vi "Firmware.vi"() -> ()   [LabVIEW 2017]
uses:
  <vilib>/Platform/TimedLoop/XDataNode/timing_clust.ctl
  <vilib>/Platform/TimedLoop/XDataNode/nitl_modes.ctl
  <vilib>/Platform/TimedLoop/XDataNode/wakeup.ctl
  <instrlib>/_niInstr/FIFO Register Bus/v1/FPGA/niInstr FIFO Register Bus v1 FPGA.lvclass
  C:/Program Files (x86)/National Instruments/LabVIEW 2017/instr.lib/_niInstr/Instruction Framework/v1/FPGA/Interfaces/Instruction Producer/Instruction Producer.lvclass
  <instrlib>/_niInstr/Instruction Framework/v1/FPGA/Helper Classes/Single Address Space Collection/Single Address Space Collection.lvclass
  C:/Program Files (x86)/National Instruments/LabVIEW 2017/instr.lib/_niInstr/Instruction Framework/v1/FPGA/Interfaces/Address Space Collection/Address Space Collection.lvclass
  <vilib>/rvi/Emulation/niFpgaGetClockAttributes.vi
  <vilib>/rvi/Emulation/niFpgaSctlEmulationGetInTimedLoop.vi
  <vilib>/rvi/Emulation/niFpgaEmulationReportErrorSimple.vi
  <userlib>/_NI FLP Library/FPGA/outsideSCTL/FlpLib Multiply Shared Instance 2.vi
  <userlib>/_NI FLP Library/FPGA/outsideSCTL/FlpLib Add Shared Instance 2.vi
  <userlib>/_NI FLP Library/FPGA/outsideSCTL/FlpLib Subtract Shared Instance 2.vi
  <userlib>/_NI FLP Library/FPGA/outsideSCTL/FlpLib Greater Than Shared Instance 2.vi
  <vilib>/rvi/Emulation/niFpgaProcessEmulError.vi
  <userlib>/_NI FLP Library/FPGA/outsideSCTL/FlpLib Cosine Shared Instance 2.vi
  <vilib>/rvi/Emulation/niFpgaCriticalErrorInLSC.vi
  <userlib>/_NI FLP Library/addons/PowerElectronics/ABCtoAlphaBeta_3PhaseUnitaryMagnitude/FlpLib ABCtoAlphaBeta_3PhaseUnitaryMagnitude 0.vi
  <userlib>/_NI FLP Library/FPGA/outsideSCTL/FlpLib Sine & Cosine Shared Instance 0.vi
  <userlib>/_NI FLP Library/addons/PowerElectronics/AlphaBetaToDQ_noSine/FlpLib AlphaBetaToDQ_noSine 0.vi
  <vilib>/platform/TimedLoop/XDataNode/XDataNode.xnode
  <vilib>/NI/PowerElectronicsControl/ThreePhasePLL/FPGA/ThreePhasePLL.lvlib
  <instrlib>/_niInstr/Instruction Framework/v1/FPGA/Top Level Bus/Register Configuration/Register Configuration.lvclass
  <vilib>/Platform/TimedLoop/XDataNode/XDNodeRunTimeDep.lvlib
  <vilib>/NI/PowerElectronicsControl/ThreePhasePLL/FPGA/AddressSpace.lvclass
panel:
  in  "fifo reg bus ctrl 0":u32
  out "fifo reg bus status 0":u32
  out "fifo reg bus data 0":u64
  in  "PLL_Timing":u32=400
  out "PLLTimingActual":u32
  out "gridFrequency":sgl
  out "freq error":sgl
  out "theta error":sgl
  in  "ThreePhaseGenTiming":u32=400
  out "ThreePhaseGenActual":u32
  in  "dTGen":sgl=1e-05 format="%#_13g"
  in  "GenFreqRadPerSec":sgl=376.991 format="%#_13g"
  out "gridTheta":sgl
  out "A":sgl
  out "B":sgl
  out "C":sgl
  in  "gain":sgl=100.0
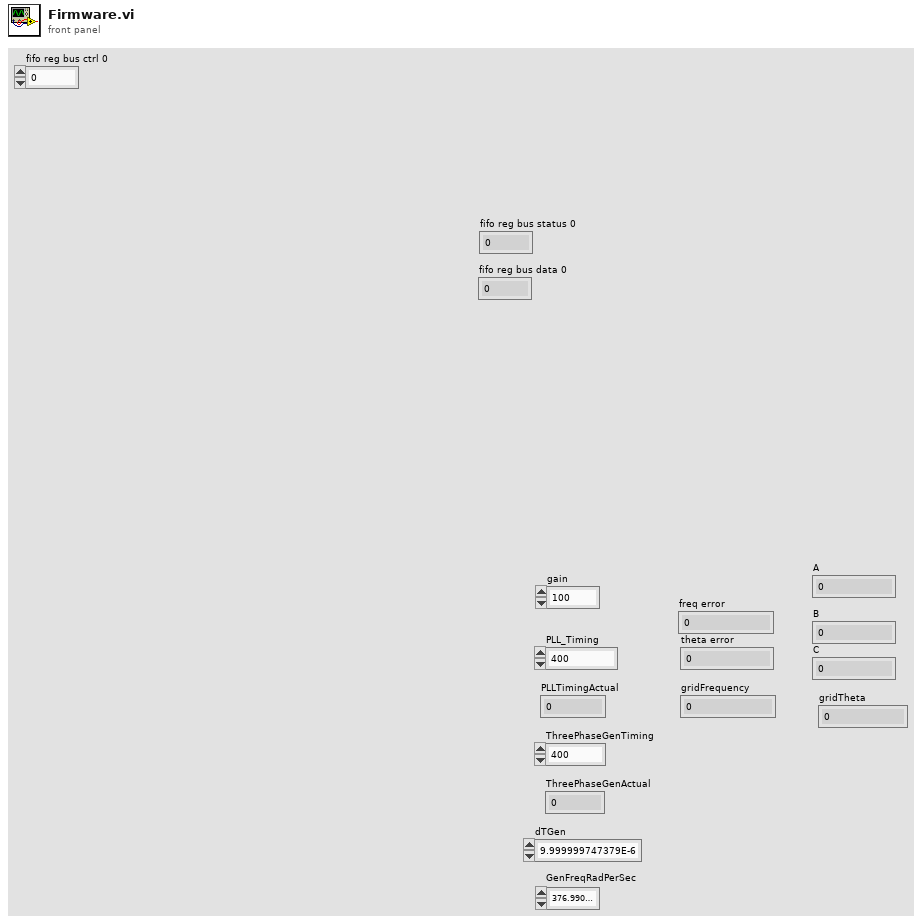
[diagram p1: front panel]
types:
  T1 = typedef "ThreePhasePLL.lvlib/registers.ctl" = cluster{"PLLGains":refnum<k21>, "PLLRange":refnum<k21>, "PLL_reset":refnum<k21>, "PLL_locked":refnum<k21>, "freqBoundaries":refnum<k21>, "expectedFreq":refnum<k21>, "lockDuration":refnum<k21>, "dT":refnum<k21>, "detectedFreq":refnum<k21>, "adjustTheta":refnum<k21>}
  T2 = typedef "XDNodeRunTimeDep.lvlib/timing_clust.ctl" = cluster{"Expected End [f-1]":u64, "Actual End [f-1]":u64, "Finished Late? [f-1]":bool, "Expected End [i-1]":u64, "Actual End [i-1]":u64, "Finished Late? [i-1]":bool, "Expected Start [i]":u64, "Actual Start [i]":u64, "Expected Start [f]":u64, "Actual Start [f]":u64, "Source Name":string, "Structure Name":string, "Period":i64, "Deadline":i64, "Offset":i64, "Start":i64, "Priority":i32, "Timeout":i32, "Mode":T3, "Wakeup Reason":T4, "Error":errorcluster, "Source Type":string, "Secondary Source Type":string, "Global End Time":u64, "Global Start Time":u64, "Frame Duration":u64, "Iteration Duration":u64, "Assigned CPU":i32, "I/O Scan Engine Mode":u32}
  T3 = typedef "XDNodeRunTimeDep.lvlib/nitl_modes.ctl" = enum32{"No Change", "Process missed periods, maintain original phase", "Discard missed periods, maintain original phase", "Process missed periods, ignore original phase", "Discard missed periods, ignore original phase"}
  T4 = typedef "XDNodeRunTimeDep.lvlib/wakeup.ctl" = enum32{"Normal", "Aborted", "Asynchronous wakeup", "Timing source error", "Timed loop error", "Timeout"}
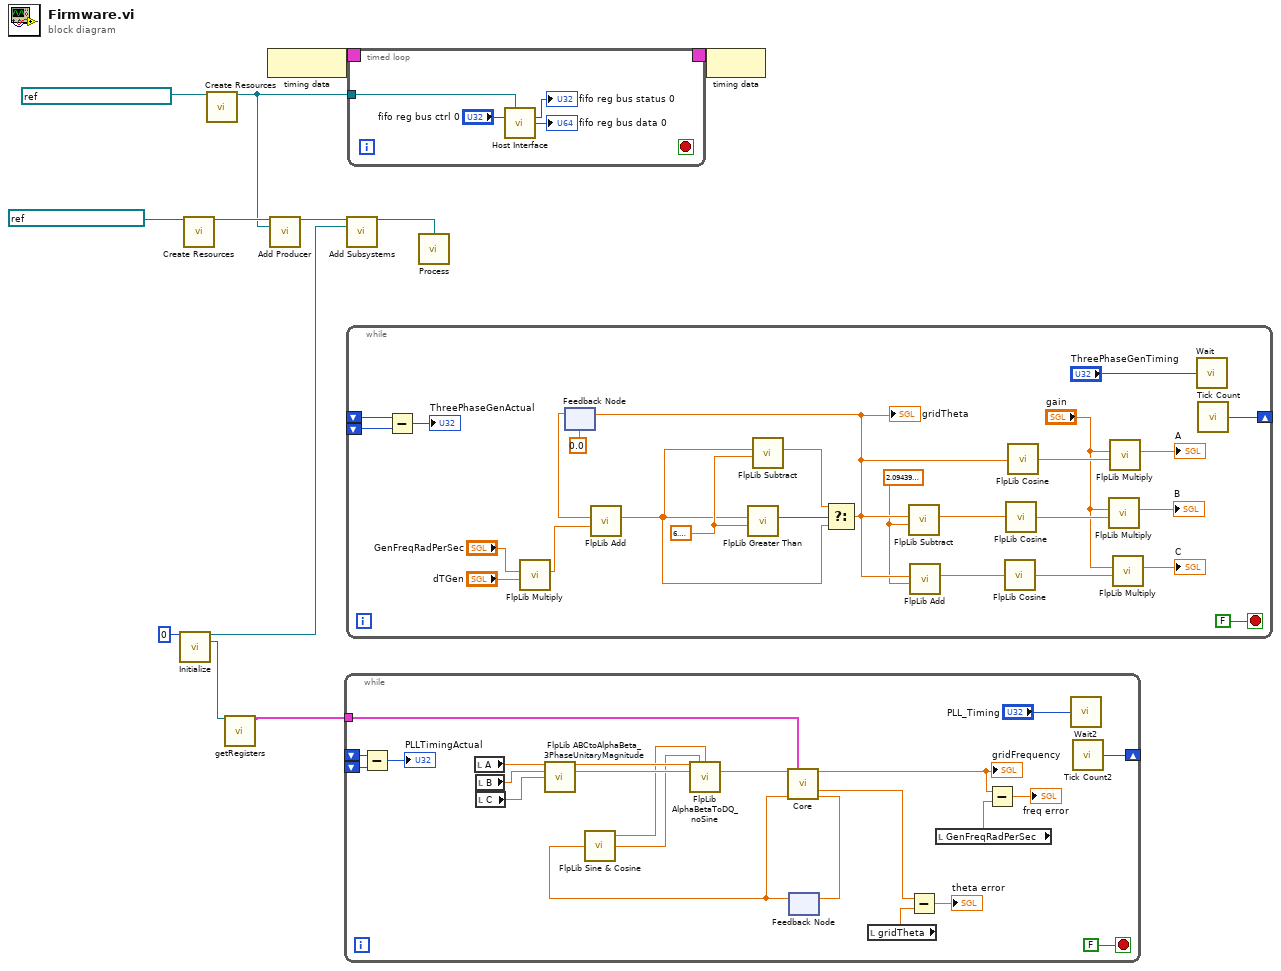
[diagram p0: block diagram]
diagram:
  n1 = call <vilib>:"Initialize.vi"("instance"=u8 0) -> ("subsysytem"=w2:refnum<class "Single Address Space Collection.lvclass">, "AddressSpace"=w4:refnum<class "AddressSpace.lvclass">)  [unwired: 13 in]
  n2 = call <instrlib>:"Create Resources.vi"("register clock"=refnum<k21> "40 MHz Onboard Clock") -> ("register configuration"=w8:refnum<class "Register Configuration.lvclass">)  [unwired: 14 in]
  n3 = call <instrlib>:"Create Resources.vi"("instruction fifo"=refnum<k21> "reg.host instruction fifo 0") -> ("fifo register bus"=w6:refnum<class "niInstr FIFO Register Bus v1 FPGA.lvclass">)  [unwired: 14 in]
  n4 = call <vilib>:"getRegisters.vi"("AddressSpace"=w4) -> ("registers"=w3:T1)  [unwired: 14 in]
  n5 = node-c288() -> (w12:T2)
  n6 = call <instrlib>:"Add Producer.vi"("register configuration in"=w8, "instruction producer"=w6) -> ("register configuration out"=w7:refnum<class "Register Configuration.lvclass">)  [unwired: 13 in]
  n7 = while {
    shift-right: [w29] -> _
    shift-left: _ -> [w28]
    shift-left: _ -> [w27]
    tunnel: w3 -> [w14]
    stop <- FALSE stop-if-true
    n8 = Subtract(x=w28, y=w27) -> (x-y=→"PLLTimingActual":u32)
    n9 = local read "A"() -> (w35:sgl)
    n10 = local read "B"() -> (w34:sgl)
    n11 = local read "C"() -> (w33:sgl)
    n12 = call-poly <userlib>:"FlpLib ABCtoAlphaBeta_3PhaseUnitaryMagnitude.vi"("A"=w35, "B"=w34, "C"=w33) -> ("alpha"=w32:sgl, "beta"=w31:sgl)  [unwired: 11 in]
    n13 = feedback #1() -> (w15:sgl)  [unwired: 1 in]
    n14 = call-poly <userlib>:"FlpLib Sine & Cosine.vi"("x"=w15) -> ("cos(x)"=w24:sgl, "sin(x)"=w23:sgl)  [unwired: 3 in]
    n15 = call-poly <userlib>:"FlpLib AlphaBetaToDQ_noSine.vi"("alpha"=w32, "cosx"=w24, "sinx"=w23, "beta"=w31) -> ("quadrature"=w18:sgl)  [unwired: 10 in, 1 out]
    n16 = call <vilib>:"Core.vi"("Vq"=w18, "registers"=w14, "ThetaIn"=w15) -> ("gridFrequency"=w17:sgl, "adjustedTheta"=w13:sgl, "ThetaOut"=w16:sgl)  [unwired: 9 in, 1 out]
    "gridFrequency" <- w17
    n17 = feedback-in #1(w16) -> ()
    n18 = local read "gridTheta"() -> (w20:sgl)
    n19 = Subtract(x=w13, y=w20) -> (x-y=→"theta error":sgl)
    n20 = local read "GenFreqRadPerSec"() -> (w22:sgl)
    n21 = Subtract(x=w17, y=w22) -> (x-y=→"freq error":sgl)
    n22 = call "Wait2"("Count(Ticks)"="PLL_Timing") -> ()  [unwired: 1 out]
    n23 = call "Tick Count2"() -> ("Tick Count(Ticks)"=w29:u32)
  }
  n24 = call <instrlib>:"Add Subsystems.vi"("register configuration in"=w7, "subsystems"=w2) -> ("register configuration out"=w5:refnum<class "Register Configuration.lvclass">)  [unwired: 13 in]
  n25 = while {
    shift-right: [w60] -> _
    shift-left: _ -> [w44]
    shift-left: _ -> [w43]
    stop <- FALSE stop-if-true
    w47 = sgl 2.0944 ("y")
    w52 = sgl 6.2831855
    n26 = Subtract(x=w44, y=w43) -> (x-y=→"ThreePhaseGenActual":u32)
    n27 = call-poly <userlib>:"FlpLib Multiply.vi"("y"="dTGen", "x"="GenFreqRadPerSec") -> ("x*y"=w54:sgl)  [unwired: 5 in]
    n28 = feedback #2(sgl 0.0) -> (w55:sgl)
    n29 = call-poly <userlib>:"FlpLib Add.vi"("y"=w54, "x"=w55) -> ("x+y"=w50:sgl)  [unwired: 5 in]
    n30 = call-poly <userlib>:"FlpLib Greater Than.vi"("y"=w52, "x"=w50) -> ("x > y?"=w53:bool)  [unwired: 5 in]
    n31 = call-poly <userlib>:"FlpLib Subtract.vi"("y"=w52, "x"=w50) -> ("x-y"=w51:sgl)  [unwired: 5 in]
    n32 = Select(t=w51, s=w53, f=w50) -> (s? t:f=w48:sgl)
    "gridTheta" <- w48
    n33 = feedback-in #2(w48) -> ()
    n34 = call-poly <userlib>:"FlpLib Subtract.vi"("y"=w47, "x"=w48) -> ("x-y"=w49:sgl)  [unwired: 5 in]
    n35 = call-poly <userlib>:"FlpLib Add.vi"("y"=w47, "x"=w48) -> ("x+y"=w46:sgl)  [unwired: 5 in]
    n36 = call-poly <userlib>:"FlpLib Cosine.vi"("x"=w46) -> ("cos(x)"=w42:sgl)  [unwired: 4 in]
    n37 = call-poly <userlib>:"FlpLib Cosine.vi"("x"=w49) -> ("cos(x)"=w41:sgl)  [unwired: 4 in]
    n38 = call-poly <userlib>:"FlpLib Cosine.vi"("x"=w48) -> ("cos(x)"=w40:sgl)  [unwired: 4 in]
    n39 = call-poly <userlib>:"FlpLib Multiply.vi"("y"=w41, "x"="gain") -> ("x*y"=→"B":sgl)  [unwired: 5 in]
    n40 = call-poly <userlib>:"FlpLib Multiply.vi"("y"=w40, "x"="gain") -> ("x*y"=→"A":sgl)  [unwired: 5 in]
    n41 = call-poly <userlib>:"FlpLib Multiply.vi"("y"=w42, "x"="gain") -> ("x*y"=→"C":sgl)  [unwired: 5 in]
    n42 = call "Wait"("Count(Ticks)"="ThreePhaseGenTiming") -> ()  [unwired: 1 out]
    n43 = call "Tick Count"() -> ("Tick Count(Ticks)"=w60:u32)
  }
  n44 = timed-loop {
    timing: w12 -> [_]
    timing-out: [_] -> w11
    tunnel: w6 -> [w65]
    stop <- _ stop-if-true
    n45 = call <instrlib>:"Host Interface.vi"("fifo register bus"=w65, "fifo reg bus ctrl 0"="fifo reg bus ctrl 0") -> ("fifo reg bus status 0"=→"fifo reg bus status 0":u32, "fifo reg bus data 0"=→"fifo reg bus data 0":u64)  [unwired: 12 in]
  }
  n46 = call <instrlib>:"Process.vi"("register configuration"=w5) -> ()  [unwired: 15 in]
  n47 = node-c288(w11) -> ()
